vi "Swerve Math.vi"(0 "Trackwidth (W)":dbl, 1 "Wheelbase (L)":dbl, 5 "Y -FWD":dbl, 7 "X1 STR":dbl, 9 "X2 RCW":dbl, 12 "Gyro Angle in degrees":dbl) -> (2 "wa3":dbl, 3 "wa4":dbl, 4 "ws1":dbl, 6 "ws2":dbl, 8 "ws3":dbl, 10 "ws4":dbl, 13 "wa2":dbl, 14 "wa1":dbl)   [LabVIEW 2023]
panel:
  # "ws1, wa1 : Front Right\nws2, wa2 : Front Left\nws3, wa3 : Back Left\nws4, wa4 : Back Right"
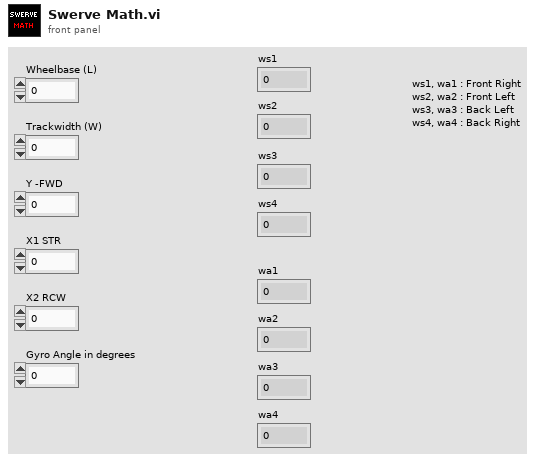
[diagram p1: front panel]
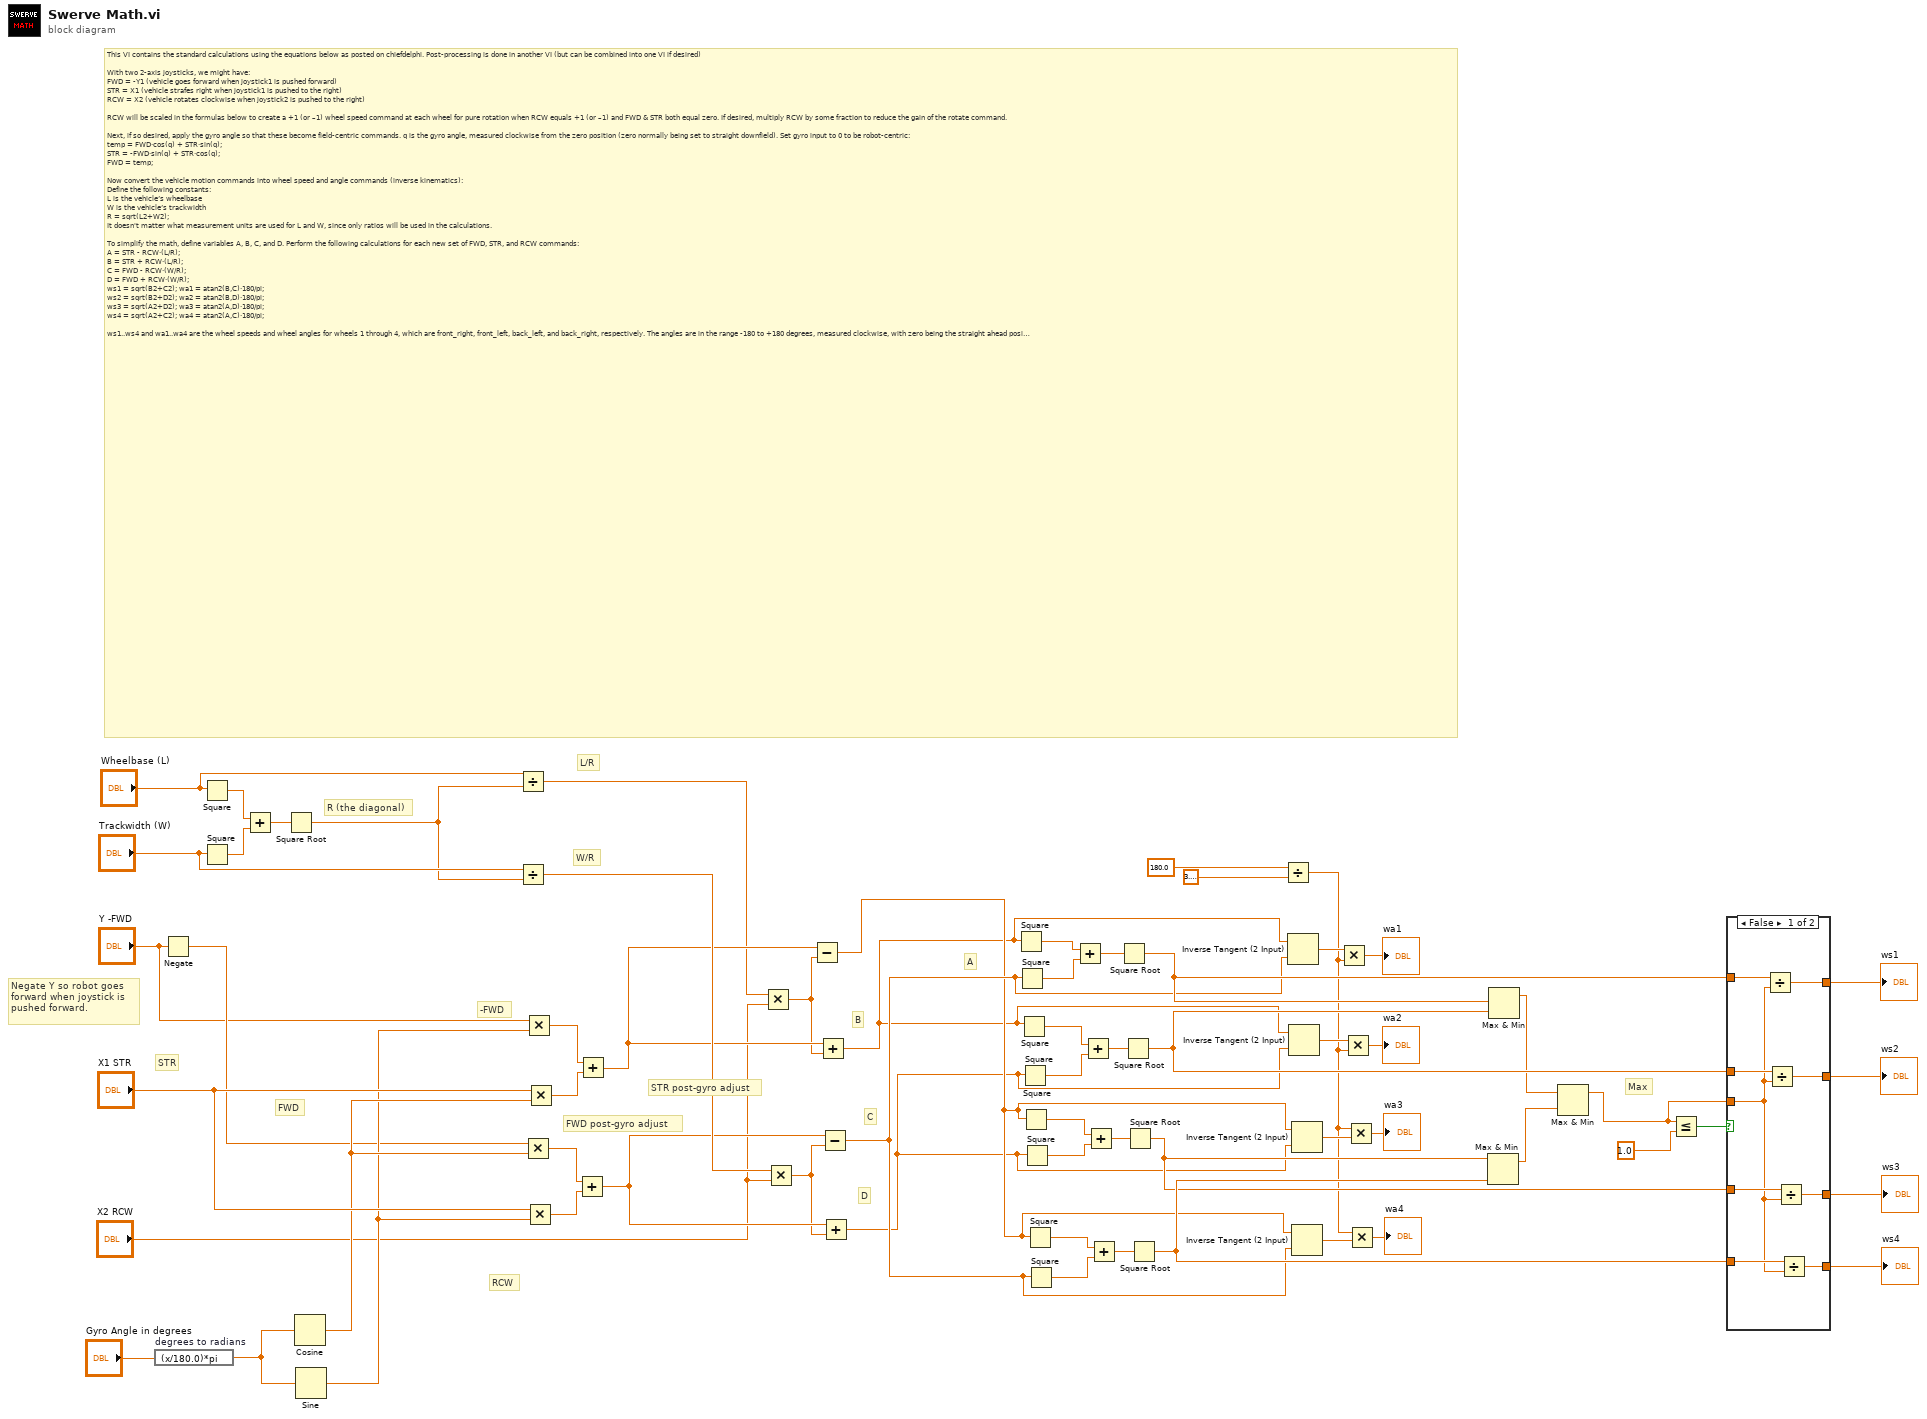
[diagram p0: block diagram]
diagram:
  # "This VI contains the standard calculations using the equations below as posted on chiefdelphi. Post-processing is done in another VI (but can be combined into one VI if desired)\n\nWith two 2-axis joysticks, we might have:\nFWD = -Y1 (vehicle goes forward when joystick1 is pushed forward)\nSTR = X1 (vehicle strafes right when joystick1 is pushed to the right)\nRCW = X2 (vehicle rotates clockwise when joystick2 is pushed to the right)\n\nRCW will be scaled in the formulas below to create a +1 (or –1) wheel speed command at each wheel for pure rotation when RCW equals +1 (or –1) and FWD & STR both equal zero. If desired, multiply RCW by some fraction to reduce the gain of the rotate command.\n\nNext, if so desired, apply the gyro angle so that these become field-centric commands. q is the gyro angle, measured clockwise from the zero position (zero normally being set to straight downfield). Set gyro input to 0 to be robot-centric:\ntemp = FWD·cos(q) + STR·sin(q);\nSTR = -FWD·sin(q) + STR·cos(q);\nFWD = temp;\n\nNow convert the vehicle motion commands into wheel speed and angle commands (inverse kinematics):\nDefine the following constants:\nL is the vehicle’s wheelbase\nW is the vehicle’s trackwidth\nR = sqrt(L2+W2);\nIt doesn't matter what measurement units are used for L and W, since only ratios will be used in the calculations.\n\nTo simplify the math, define variables A, B, C, and D. Perform the following calculations for each new set of FWD, STR, and RCW commands:\nA = STR - RCW·(L/R);\nB = STR + RCW·(L/R);\nC = FWD - RCW·(W/R);\nD = FWD + RCW·(W/R);\nws1 = sqrt(B2+C2); wa1 = atan2(B,C)·180/pi;\nws2 = sqrt(B2+D2); wa2 = atan2(B,D)·180/pi;\nws3 = sqrt(A2+D2); wa3 = atan2(A,D)·180/pi;\nws4 = sqrt(A2+C2); wa4 = atan2(A,C)·180/pi;\n\nws1..ws4 and wa1..wa4 are the wheel speeds and wheel angles for wheels 1 through 4, which are front_right, front_left, back_left, and back_right, respectively. The angles are in the range -180 to +180 degrees, measured clockwise, with zero being the straight ahead position. The wheel speeds need to be normalized before being used, as follows:\nmax = the largest of ws1, ws2, ws3, ws4 \nif (max >1) {ws1/=max; ws2/=max; ws3/=max; ws4/=max;} \n\nThe 4 wheel speeds are now in the range 0 to +1. Notice 0 to +1 and not -1 to +1, because each speed is always in the direction of the corresponding wheel angle. The 4 wheel speed and wheel angle pairs are now suitable for sending to a control algorithm which will decide how to actuate the steering and drive motors to achieve those speeds and angles for each wheel.\n\nThis is a separate and interesting problem, which may involve, for example, logic to reverse the wheel speed instead of steering the wheel 180 degrees (and similarly for other steering/speed commands). This control logic is highly dependent on the limitations of the vehicle design, such as the response of the steering motor, and the fact that some vehicles may have limitless steering (coaxial or slip rings) whereas others may be steering-limited. More complex logic may also take into account the current vehicle speed and recent past history in innovative ways. Computing the necessary speed and angle errors to send to a PID control (for example) may therefore become a non-trivial task in an effort to achieve smooth and seamless control."
  # "-FWD"
  # "Negate Y so robot goes\nforward when joystick is\npushed forward."
  # "Max"
  # "A"
  # "B"
  # "C"
  # "D"
  # "STR post-gyro adjust"
  # "FWD post-gyro adjust"
  # "RCW"
  # "STR"
  # "FWD"
  # "R (the diagonal)"
  # "W/R"
  # "L/R"
  n1 = expression code="(x/180.0)*pi" "degrees to radians"("Gyro Angle in degrees") -> (w5:dbl)
  n2 = Negate(x="Y -FWD") -> (-x=w15:dbl)
  n3 = Square(x="Wheelbase (L)") -> (x^2=w8:dbl)
  n4 = Square(x="Trackwidth (W)") -> (x^2=w9:dbl)
  n5 = Add(x=w8, y=w9) -> (x+y=w10:dbl)
  n6 = Square Root(x=w10) -> (sqrt(x)=w7:dbl)
  n7 = Cosine(x=w5) -> (cos(x)=w17:dbl)
  n8 = Sine(x=w5) -> (sin(x)=w16:dbl)
  n9 = Divide(x="Wheelbase (L)", y=w7) -> (x/y=w21:dbl)
  n10 = Divide(x="Trackwidth (W)", y=w7) -> (x/y=w24:dbl)
  n11 = Multiply(x=w15, y=w17) -> (x*y=w11:dbl)
  n12 = Multiply(x="Y -FWD", y=w16) -> (x*y=w13:dbl)
  n13 = Multiply(x="X1 STR", y=w16) -> (x*y=w12:dbl)
  n14 = Multiply(x="X1 STR", y=w17) -> (x*y=w14:dbl)
  n15 = Add(x=w11, y=w12) -> (x+y=w23:dbl)
  n16 = Add(x=w13, y=w14) -> (x+y=w22:dbl)
  n17 = Multiply(x=w21, y="X2 RCW") -> (x*y=w3:dbl)
  n18 = Multiply(x=w24, y="X2 RCW") -> (x*y=w2:dbl)
  n19 = Subtract(x=w22, y=w3) -> (x-y=w50:dbl)
  n20 = Add(x=w22, y=w3) -> (x+y=w48:dbl)
  n21 = Subtract(x=w23, y=w2) -> (x-y=w51:dbl)
  n22 = Add(x=w23, y=w2) -> (x+y=w49:dbl)
  n23 = Square(x=w48) -> (x^2=w29:dbl)
  n24 = Square(x=w51) -> (x^2=w30:dbl)
  n25 = Square(x=w48) -> (x^2=w31:dbl)
  n26 = Square(x=w49) -> (x^2=w32:dbl)
  n27 = Square(x=w50) -> (x^2=w33:dbl)
  n28 = Square(x=w49) -> (x^2=w34:dbl)
  n29 = Square(x=w50) -> (x^2=w35:dbl)
  n30 = Square(x=w51) -> (x^2=w36:dbl)
  n31 = Add(x=w29, y=w30) -> (x+y=w25:dbl)
  n32 = Add(x=w31, y=w32) -> (x+y=w26:dbl)
  n33 = Add(x=w33, y=w34) -> (x+y=w27:dbl)
  n34 = Add(x=w35, y=w36) -> (x+y=w28:dbl)
  n35 = Square Root(x=w25) -> (sqrt(x)=w56:dbl)
  n36 = Square Root(x=w26) -> (sqrt(x)=w57:dbl)
  n37 = Square Root(x=w27) -> (sqrt(x)=w58:dbl)
  n38 = Square Root(x=w28) -> (sqrt(x)=w59:dbl)
  n39 = Divide(x=180.0, y=3.141592653589793) -> (x/y=w43:dbl)
  n40 = Inverse Tangent (2 Input)(1:w51, 2:w48) -> (0:w47:dbl)
  n41 = Inverse Tangent (2 Input)(1:w49, 2:w48) -> (0:w46:dbl)
  n42 = Inverse Tangent (2 Input)(1:w49, 2:w50) -> (0:w45:dbl)
  n43 = Inverse Tangent (2 Input)(1:w51, 2:w50) -> (0:w44:dbl)
  n44 = Multiply(x=w47, y=w43) -> (x*y=→"wa1":dbl)
  n45 = Multiply(x=w46, y=w43) -> (x*y=→"wa2":dbl)
  n46 = Multiply(x=w43, y=w45) -> (x*y=→"wa3":dbl)
  n47 = Multiply(x=w43, y=w44) -> (x*y=→"wa4":dbl)
  n48 = Max & Min(x=w58, y=w59) -> (max(x,y)=w52:dbl)  [unwired: 1 out]
  n49 = Max & Min(x=w56, y=w57) -> (max(x,y)=w53:dbl)  [unwired: 1 out]
  n50 = Max & Min(x=w53, y=w52) -> (max(x,y)=w60:dbl)  [unwired: 1 out]
  n51 = Less Or Equal?(x=w60, y=1.0) -> (x <= y?=w54:bool)
  n52 = case shown="False" w54 {
    tunnel: w56 -> [w70 w77]
    tunnel: w57 -> [w71 w76]
    tunnel: w58 -> [w73 w75]
    tunnel: w59 -> [w72 w74]
    tunnel: w60 -> [w69 _]
    tunnel: [w68 w77] -> w61
    tunnel: [w67 w76] -> w62
    tunnel: [w66 w75] -> w63
    tunnel: [w65 w74] -> w64
    frame False {
      n53 = Divide(x=w70, y=w69) -> (x/y=w68:dbl)
      n54 = Divide(x=w71, y=w69) -> (x/y=w67:dbl)
      n55 = Divide(x=w73, y=w69) -> (x/y=w66:dbl)
      n56 = Divide(x=w72, y=w69) -> (x/y=w65:dbl)
    }
    frame True {
    }
  }
  "ws4" <- w64
  "ws3" <- w63
  "ws2" <- w62
  "ws1" <- w61
